vi "Path.vi"(8 "error in":errorcluster, 11 "Path in":refnum<vi>) -> (0 "error out":errorcluster, 3 "Path out":refnum<class "Path.lvclass">)   [LabVIEW 2014, in "Raspberry Pi Compatible Compiler for LabVIEW.lvlib" / "Path.lvclass"]
uses:
  Path.lvclass
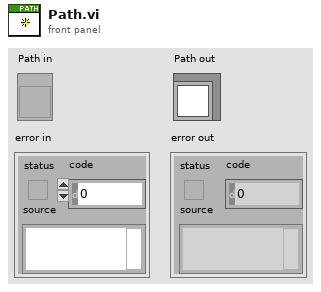
[diagram p1: front panel]
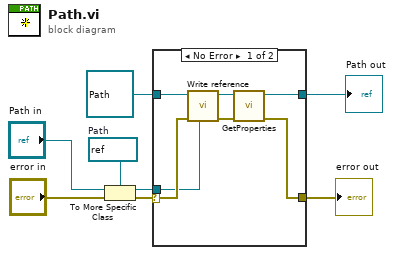
[diagram p0: block diagram]
diagram:
  w6 = refnum<vi> refnum  # Path
  n1 = To More Specific Class(target class=w6, reference="Path in", error in="error in") -> (specific class reference=w4:refnum<vi>, error out=w5:errorcluster)
  n2 = case shown="No Error" w5 {
    selector: w5 -> [w15 w17]
    tunnel: w4 -> [w13 _]
    tunnel: refnum<class "Path.lvclass"> refnum ("Path in") -> [w14 w16]
    tunnel: [w10 w16] -> w2
    tunnel: [w9 w17] -> w1
    frame No Error {
      n3 = call-dynamic "Write reference.vi"("reference"=w13, "error in"=w15, "GObject in"=w14) -> ("error out"=w11:errorcluster, "GObject out"=w12:refnum<class "Path.lvclass">)  [unwired: 5 in]
      n4 = call-dynamic "GetProperties.vi"("error in"=w11, "Path in"=w12) -> ("error out"=w9:errorcluster, "Path out"=w10:refnum<class "Path.lvclass">)  [unwired: 8 in]
    }
    frame Error {
    }
  }
  "error out" <- w1
  "Path out" <- w2
